vi "AO SCTR Stop If Running.vi"(0 "AO SCTR Notifier":refnum<notifier>) -> (4 "AO SCTR Notifier (Dup)":refnum<notifier>, 15 "Latest Notification":T1={"Actions"=enum."Stop at Offset", "Offset (V)"=-0.159, "Amplititude (V)"=0.524, "Samples Per Channel"=225, "Start Delay (ms)"=10.0, "Running?"=FALSE, "Exposure Time (s)"=0.0} {"Amplititude (V)" format="%#_13g"; "Offset (V)" format="%#_13g"; "Start Delay (ms)" format="%#_13g"})   [LabVIEW 2021]
uses:
  AO SCTR Type Defs/AO SCTR Notifier Type.ctl
  AO SCTR Type Defs/AO SCTR Actions.ctl
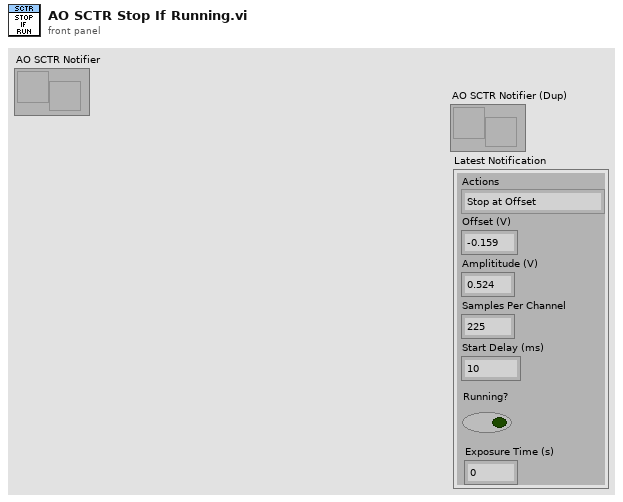
[diagram p1: front panel]
types:
  T1 = typedef "AO SCTR Notifier Type.ctl" = cluster{"Actions":T2, "Offset (V)":dbl, "Amplititude (V)":dbl, "Samples Per Channel":i32, "Start Delay (ms)":dbl, "Running?":bool, "Exposure Time (s)":dbl}
  T2 = typedef "AO SCTR Actions.ctl" = enum16{"Stop at Offset", "Update and Run", "Quit"}
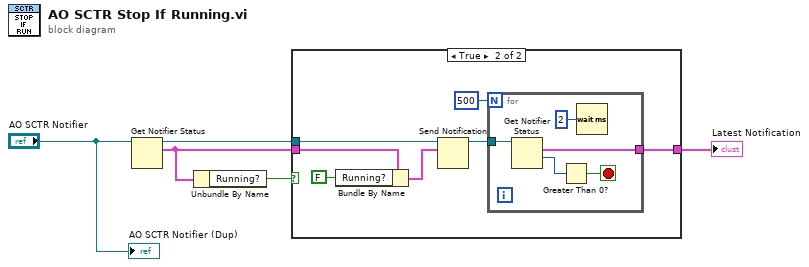
[diagram p0: block diagram]
diagram:
  n1 = Get Notifier Status(notifier="AO SCTR Notifier") -> (notifier out=w4:refnum<notifier>, current notification=w3:T1)  [unwired: 1 in, 3 out]
  n2 = Unbundle By Name(w3) -> ("Running?"=w5:bool)
  n3 = case shown="True" w5 {
    tunnel: w4 -> [_ w13]
    tunnel: w3 -> [w6 w11]
    tunnel: [w6 w8] -> w1
    frame False {
    }
    frame True {
      n4 = Bundle By Name(cluster=w11, "Running?"=FALSE) -> (w9:T1)
      n5 = Send Notification(notification=w9, notifier=w13) -> (notifier out=w12:refnum<notifier>)  [unwired: 1 in, 1 out]
      n6 = for {
        N: 500 -> [_]
        tunnel: w12 -> [w18]
        tunnel: [w15] -> w8
        stop <- w14 stop-if-true
        n7 = Get Notifier Status(notifier=w18) -> (current notification=w15:T1, # waiting=w16:i32)  [unwired: 1 in, 3 out]
        n8 = Greater Than 0?(x=w16) -> (x > 0?=w14:bool)
        n9 = Wait (ms)(milliseconds to wait=u32 2) -> ()  [unwired: 1 out]
      }
    }
  }
  "Latest Notification" <- w1
  "AO SCTR Notifier (Dup)" <- "AO SCTR Notifier"
